vi "While_Sum.vi"() -> ()   [LabVIEW 2024]
panel:
  out "Numeric 2":i32
  in  "Numeric":dbl
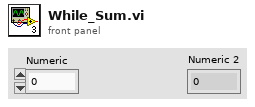
[diagram p1: front panel]
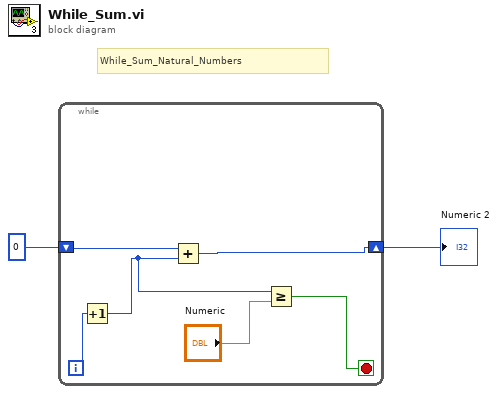
[diagram p0: block diagram]
diagram:
  # "While_Sum_Natural_Numbers"
  n1 = while {
    shift-right: [w6] -> w1
    shift-left: 0 -> [w5]
    i -> [w4]
    stop <- w7 stop-if-true
    n2 = Increment(x=w4) -> (x+1=w3:i32)
    n3 = Add(x=w5, y=w3) -> (x+y=w6:i32)
    n4 = Greater Or Equal?(x=w3, y="Numeric") -> (x >= y?=w7:bool)
  }
  "Numeric 2" <- w1
